vi "read2Byte Rx.vi"(10 "protocol_version":i32, 11 "port_num":i32) -> (3 "function return":u16)   [LabVIEW 2021, in "dxl_x86_c.lvlib"]
doc: "WINDECLSPEC uint16_t read2ByteRx (int port_num, int protocol_version);"
uses:
  dxl_x86_c.lvlib
  dxl_x86_c.dll
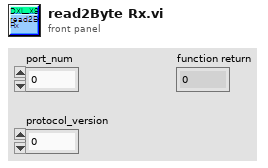
[diagram p1: front panel]
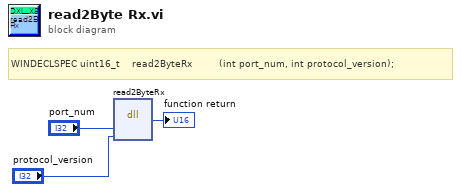
[diagram p0: block diagram]
diagram:
  # "WINDECLSPEC uint16_t    read2ByteRx         (int port_num, int protocol_version);"
  n1 = dll-call lib="C:/Users/ashek/Desktop/ashekim/ws/DynamixelSDK/labview/labview/dxl_x86_c.*" fn="read2ByteRx"("port_num"="port_num", "protocol_version"="protocol_version") -> (→"function return":u16)  [unwired: 5 in, 2 out]
